vi "Get Parameter.vi"(8 "error in (no error)":errorcluster caption="entrée d'erreur (pas d'erreur)", 11 "P2056_Send_Command_UART en entrée":refnum<class "P2056_Send_Command_UART.lvclass">) -> (0 "error out":errorcluster caption="sortie d'erreur", 2 "Parameter":string, 3 "P2056_Send_Command_UART en sortie":refnum<class "P2056_Send_Command_UART.lvclass">)   [LabVIEW 2020, in "Library Test.lvlib" / "P2056_Send_Command_UART.lvclass"]
uses:
  P2056_Send_Command_UART.lvclass
  P2056_Send_Command_UART.lvclass/P2056_Send_Command_UART.ctl
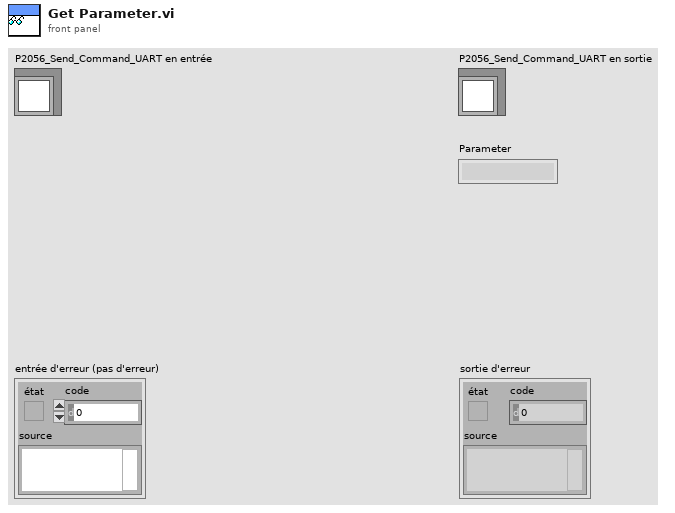
[diagram p1: front panel]
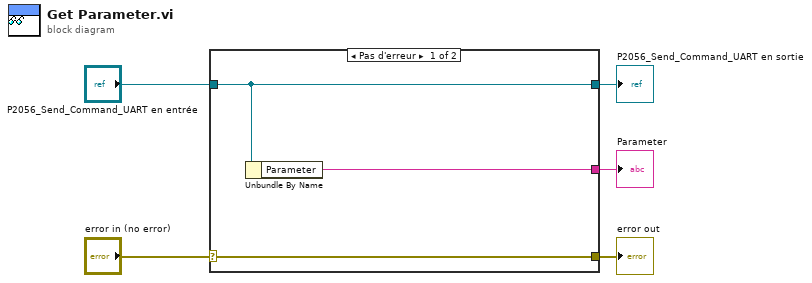
[diagram p0: block diagram]
diagram:
  n1 = case shown="Pas d'erreur" "error in (no error)" {
    selector: "error in (no error)" -> [w8 w9]
    tunnel: [w8 w9] -> w4
    tunnel: [w7 w10] -> w2
    tunnel: "P2056_Send_Command_UART en entrée" -> [w7 w10]
    tunnel: [w6 _] -> w1
    frame No Error {
      n2 = Unbundle By Name(w7) -> ("Parameter"=w6:string)
    }
    frame Error {
    }
  }
  "error out" <- w4
  "P2056_Send_Command_UART en sortie" <- w2
  "Parameter" <- w1
